vi "Wait For Acquisition By Handle Time Out.vi"(10 "iTimeOutMs":i32, 11 "cameraHandle":i32) -> (3 "function return":u32)   [LabVIEW 2018, in "Copy of Andor SDK.lvlib"]
doc: "EXPNETTYPE unsigned int WINAPI WaitForAcquisitionByHandleTimeOut(long cameraHandle, int iTimeOutMs);"
uses:
  Copy of Andor SDK.lvlib
  <userlib>/Andor SDK/ATMCD32D.dll
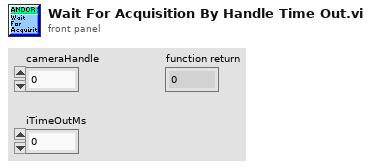
[diagram p1: front panel]
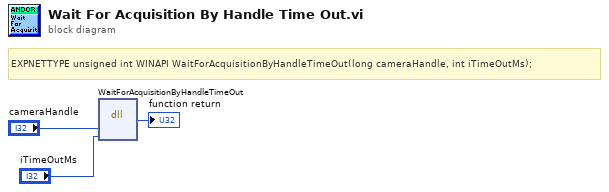
[diagram p0: block diagram]
diagram:
  # "EXPNETTYPE unsigned int WINAPI WaitForAcquisitionByHandleTimeOut(long cameraHandle, int iTimeOutMs);"
  n1 = dll-call lib="C:/Program Files (x86)/National Instruments/LabVIEW 2018/user.lib/Andor SDK/ATMCD32D.*" fn="WaitForAcquisitionByHandleTimeOut"("cameraHandle"="cameraHandle", "iTimeOutMs"="iTimeOutMs") -> (→"function return":u32)  [unwired: 5 in, 2 out]
